vi "Test Server.vi"() -> ()   [LabVIEW 2013]
uses:
  Control Packets/ControlPacket/Control Packet Type -- enum.ctl
  Connection/TCPConnection.lvclass
  Server class/Server.lvclass
  Control Packets/CONNECT/CONNECT.lvclass
  Control Packets/ControlPacket/ControlPacket.lvclass
  Control Packets/DISCONNECT/DISCONNECT.lvclass
panel:
  out "Control Packet Type":T1
  out "error out":errorcluster
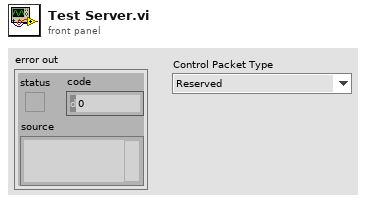
[diagram p1: front panel]
types:
  T1 = typedef "ControlPacket.lvclass/Control Packet Type -- enum.ctl" = enum16{"Reserved", "CONNECT", "CONNACK", "PUBLISH", "PUBACK", "PUBREC", "PUBREL", "PUBCOMP", "SUBSCRIBE", "SUBACK", "UNSUBSCRIBE", "UNSUBACK", "PINGREQ", "PINGRESP", "DISCONNECT", "Reserved(15)"}
  T2 = enum16{"Standard", "Buffered", "CRLF", "Immediate"}
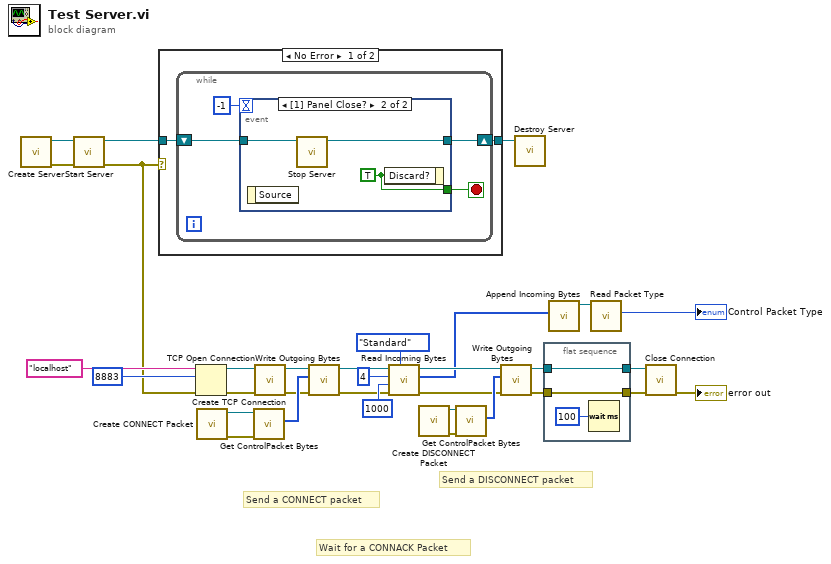
[diagram p0: block diagram]
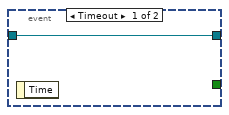
[diagram p2: hidden frame]
diagram:
  # "Wait for a CONNACK Packet"
  # "Send a DISCONNECT packet"
  # "Send a CONNECT packet"
  n1 = call "Create Server.vi"() -> ("error out"=w29:errorcluster, "Server"=w32:refnum<class "Server.lvclass">)  [unwired: 10 in]
  n2 = call "Start Server.vi"("error in (no error)"=w29, "Server in"=w32) -> ("error out"=w20:errorcluster, "Server out"=w31:refnum<class "Server.lvclass">)  [unwired: 8 in]
  n3 = case shown="No Error" w20 {
    tunnel: w31 -> [w34 w43]
    tunnel: [w33 w43] -> w30
    frame No Error {
      n4 = while {
        shift-right: [w35] -> w33
        shift-left: w34 -> [w37]
        stop <- w36 stop-if-true
        n5 = event shown="[1] Panel Close?" {
          selector: _ -> [_ _]
          dyn-events: _ -> [_ _]
          timeout: -1 -> [_ _]
          tunnel: w37 -> [w39 w42]
          tunnel: [_ w41] -> w36
          tunnel: [w39 w40] -> w35
          event Timeout {
            n6 = event-data() -> ()  [unwired: 1 in, 1 out]
          }
          event Panel Close? {
            w41 = TRUE ("Discard?")
            n7 = event-data() -> ()  [unwired: 1 in, 1 out]
            n8 = call "Stop Server.vi"("Server in"=w42) -> ("Server out"=w40:refnum<class "Server.lvclass">)  [unwired: 9 in, 1 out]
            n9 = event-data("Discard?"=w41) -> ()  [unwired: 1 in, 1 out]
          }
        }
      }
    }
    frame Error {
    }
  }
  n10 = TCP Open Connection(address="localhost", remote port or service name=u16 8883, error in (no error)=w20) -> (connection ID=w19:refnum<k5>, error out=w2:errorcluster)  [unwired: 2 in]
  n11 = call "Create CONNECT Packet.vi"() -> ("error out"=w25:errorcluster, "CONNECT"=w26:refnum<class "CONNECT.lvclass">)  [unwired: 10 in]
  n12 = call "Get ControlPacket Bytes.vi"("error in (no error)"=w25, "ControlPacket"=w26) -> ("Bytes Stream"=w17:u8[])  [unwired: 7 in, 2 out]
  n13 = call "Create TCP Connection.vi"("error in (no error)"=w2, "connection ID"=w19) -> ("error out"=w8:errorcluster, "TCPConnection out"=w18:refnum<class "TCPConnection.lvclass">)  [unwired: 8 in]
  n14 = call "Write Outgoing Bytes.vi"("error in (no error)"=w8, "Bytes"=w17, "TCPConnection in"=w18) -> ("error out"=w7:errorcluster, "TCPConnection out"=w16:refnum<class "TCPConnection.lvclass">)  [unwired: 7 in]
  n15 = call "Read Incoming Bytes.vi"("mode (standard)"=T2."Standard", "error in (no error)"=w7, "timeout (1000 ms)"=1000 ("timeout ms (25000)"), "bytes to read (100)"=4 ("bytes to read"), "TCPConnection in"=w16) -> ("error out"=w6:errorcluster, "Bytes"=w11:u8[], "TCPConnection out"=w13:refnum<class "TCPConnection.lvclass">)  [unwired: 3 in, 1 out]
  n16 = call "Create DISCONNECT Packet.vi"() -> ("error out"=w24:errorcluster, "DISCONNECT"=w23:refnum<class "DISCONNECT.lvclass">)  [unwired: 10 in]
  n17 = call "Get ControlPacket Bytes.vi"("error in (no error)"=w24, "ControlPacket"=w23) -> ("Bytes Stream"=w12:u8[])  [unwired: 7 in, 2 out]
  n18 = call "Write Outgoing Bytes.vi"("error in (no error)"=w6, "Bytes"=w12, "TCPConnection in"=w13) -> ("error out"=w4:errorcluster, "TCPConnection out"=w10:refnum<class "TCPConnection.lvclass">)  [unwired: 7 in]
  n19 = call "Destroy Server.vi"("Server in"=w30) -> ()  [unwired: 9 in, 2 out]
  n20 = flat-sequence {
    tunnel: w10 -> [w46]
    tunnel: [w46] -> w9
    tunnel: [w44] -> w5
    tunnel: w4 -> [w44]
    frame #0 {
      n21 = Wait (ms)(milliseconds to wait=u32 100) -> ()  [unwired: 1 out]
    }
  }
  n22 = call "Append Incoming Bytes.vi"("Incoming Packets"=w11) -> ("ControlPacket"=w22:refnum<class "ControlPacket.lvclass">)  [unwired: 7 in, 3 out]
  n23 = call "Read Packet Type.vi"("ControlPacket in"=w22) -> ("Control Packet Type"=→"Control Packet Type":T1)  [unwired: 9 in, 1 out]
  n24 = call-dynamic "Close Connection.vi"("error in (no error)"=w5, "TCPConnection in"=w9) -> ("error out"=→"error out":errorcluster)  [unwired: 8 in, 1 out]
